vi "State Elapsed Time.vi"(8 "error in (no error)":errorcluster, 10 "Reset (F)":bool caption="Reset", 11 "Turbo in":refnum<class "Turbo.lvclass">) -> (0 "error out":errorcluster, 1 "State Timeout?":bool caption="Time has Elapsed", 2 "Elapsed Time (s)":dbl, 3 "Turbo out":refnum<class "Turbo.lvclass">)   [LabVIEW 2015, in "cRIO-Carbondioxide.lvlib" / "CO2-Actor.lvlib" / "Turbo.lvclass"]
uses:
  Turbo.lvclass
  Turbo.lvclass/Turbo.ctl
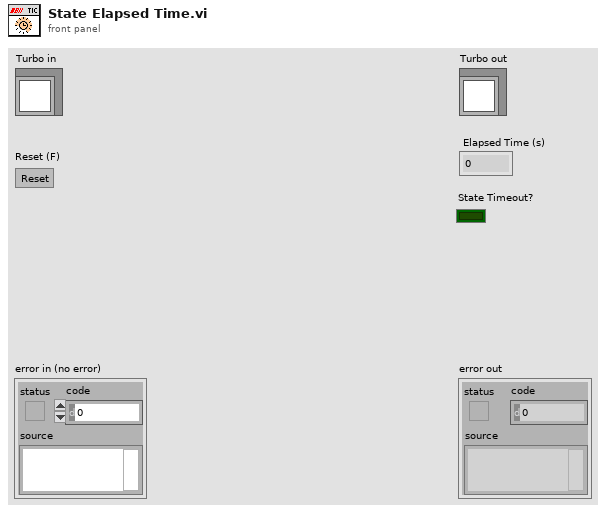
[diagram p1: front panel]
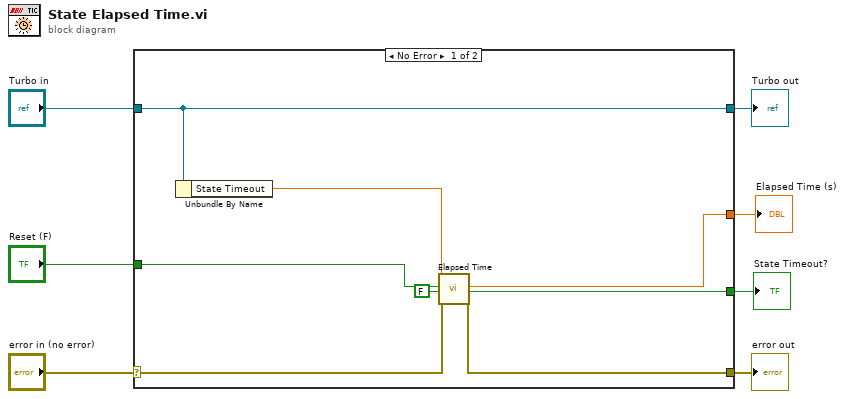
[diagram p0: block diagram]
diagram:
  n1 = case shown="No Error" "error in (no error)" {
    selector: "error in (no error)" -> [w14 w17]
    tunnel: [w13 w17] -> w6
    tunnel: [w9 w16] -> w4
    tunnel: "Turbo in" -> [w9 w16]
    tunnel: [w12 _] -> w3
    tunnel: [w10 _] -> w2
    tunnel: "Reset (F)" -> [w8 _]
    frame No Error {
      n2 = Unbundle By Name(w9) -> ("State Timeout"=w15:dbl)
      n3 = call "Elapsed Time"("Time Target (s)"=w15, "Reset"=w8, "Auto Reset"=FALSE, "error in (no error)"=w14) -> ("Elapsed Time (s)"=w10:dbl, "Time has Elapsed"=w12:bool, "error out"=w13:errorcluster)  [unwired: 8 in, 5 out]
    }
    frame Error {
    }
  }
  "error out" <- w6
  "Turbo out" <- w4
  "State Timeout?" <- w3
  "Elapsed Time (s)" <- w2
